vi "MNISTImgGenRGBSeq_sub.vi"(5 "1stRow(i)":i32, 6 "배열":i64[][](array[numeric]), 7 "BatchNum":i32=10) -> (0 "Y(RGB)":i16[](array[numeric]), 1 "2D(29_28)B":i32[][](array[numeric]), 2 "2D(29_28)G":i32[][](array[numeric]), 3 "2D(29_28)R":i32[][](array[numeric]))   [LabVIEW 2021]
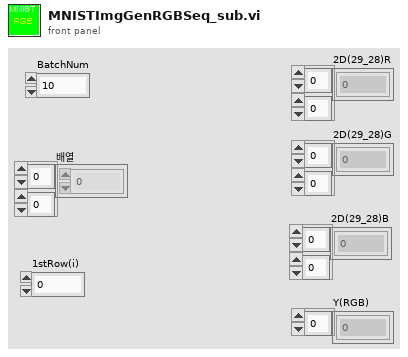
[diagram p1: front panel]
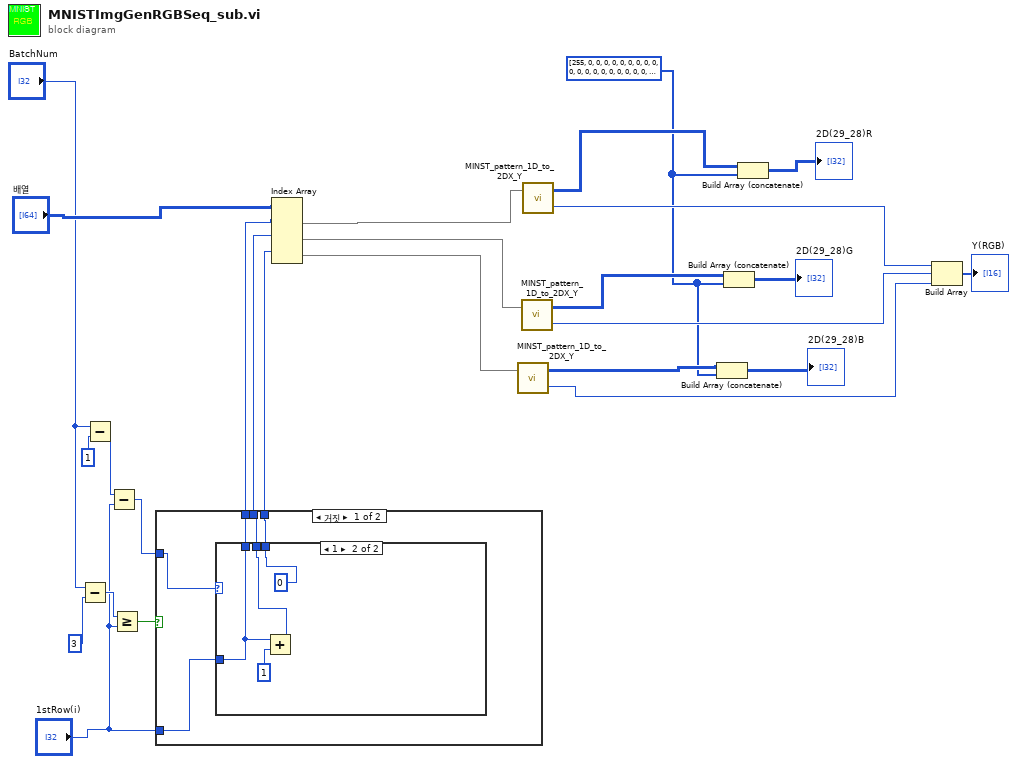
[diagram p0: block diagram]
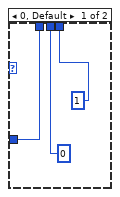
[diagram p2: hidden frame]
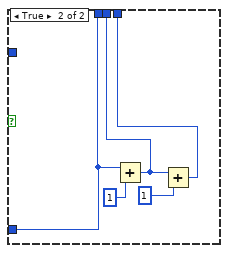
[diagram p3: hidden frame]
diagram:
  w1 = i32[] [255, 0, 0, 0, 0, 0, 0, 0, 0, 0, 0, 0, 0, 0, 0, 0, 0, 0, 0, 0, 0, 0, 0, 0, 0, 0, 0, 0] ("두 번째 부분배열")
  n1 = Subtract(x="BatchNum", y=3) -> (x-y=w20:i32)
  n2 = Subtract(x="BatchNum", y=1) -> (x-y=w18:i32)
  n3 = Subtract(x=w18, y="1stRow(i)") -> (x-y=w17:i32)
  n4 = Greater Or Equal?(x=w20, y="1stRow(i)") -> (x >= y?=w21:bool)
  n5 = case shown="거짓" w21 {
    tunnel: "1stRow(i)" -> [w30 w39]
    tunnel: [w29 w39] -> w25
    tunnel: [w28 w41] -> w24
    tunnel: [w27 w40] -> w23
    tunnel: w17 -> [w31 _]
    frame False {
      n6 = case shown="1" w31 {
        tunnel: w30 -> [w34 w38]
        tunnel: [w34 w38] -> w29
        tunnel: [0 w36] -> w28
        tunnel: [1 0 ("y")] -> w27
        frame 0, Default {
        }
        frame 1 {
          n7 = Add(x=w38, y=1) -> (x+y=w36:i32)
        }
      }
    }
    frame True {
      n8 = Add(x=w39, y=1) -> (x+y=w41:i32)
      n9 = Add(x=w41, y=1) -> (x+y=w40:i32)
    }
  }
  n10 = Index Array(array="배열", index (row) #1=w25, index (row) #2=w24, index (row) #3=w23) -> (element #1=w26:i64[], element #2=w13:i64[], element #3=w12:i64[])  [unwired: 3 in]
  n11 = call "MINST_pattern_1D_to_2DX_Y.vi"("pattern 1D"=w12) -> ("Pattern_Y"=w9:i16, "2D(28_28)"=w2:i32[][])  [unwired: 1 in]
  n12 = call "MINST_pattern_1D_to_2DX_Y.vi"("pattern 1D"=w13) -> ("Pattern_Y"=w10:i16, "2D(28_28)"=w4:i32[][])  [unwired: 1 in]
  n13 = call "MINST_pattern_1D_to_2DX_Y.vi"("pattern 1D"=w26) -> ("Pattern_Y"=w11:i16, "2D(28_28)"=w7:i32[][])  [unwired: 1 in]
  n14 = Build Array (concatenate)(w2, w1) -> (→"2D(29_28)B":i32[][])
  n15 = Build Array (concatenate)(w4, w1) -> (→"2D(29_28)G":i32[][])
  n16 = Build Array (concatenate)(w7, w1) -> (→"2D(29_28)R":i32[][])
  n17 = Build Array(w11, w10, w9) -> (→"Y(RGB)":i16[])
